vi "Untitled 1.vi"() -> ()   [LabVIEW 2018]
panel:
  in  "XYZAER":T1(array[cluster]) {"r" format="%1_6f"; "e" format="%1_6f"; "a" format="%1_6f"; "z" format="%1_6f"; "y" format="%1_6f"; "x" format="%1_6f"}
  out "Position Sensor Data":cluster{dbl, "x":sgl}[](graph)
  out "Tracker 1 - X,Y,Z":cluster{"x":sgl, "y":sgl, "z":sgl}(graph)
  out "Tracker 2 - X,Y,Z":cluster{"x":sgl, "y":sgl, "z":sgl}(graph)
  out "Tracker 3 - X,Y,Z":cluster{"x":sgl, "y":sgl, "z":sgl}(graph)
  out "Tracker 4 - X,Y,Z":cluster{"x":sgl, "y":sgl, "z":sgl}(graph)
  out "Connected":bool
  out "Start Time Text":string
  out "Stop Time Text":string
  out "Elapsed Time Text":string
  out "HostFrameCount":u32
  out "Running":bool
  out "Loop Iter":i32
  out "PnoData":bool
  in  "stop":bool
  out "error out":errorcluster {"code" format="%.0x"}
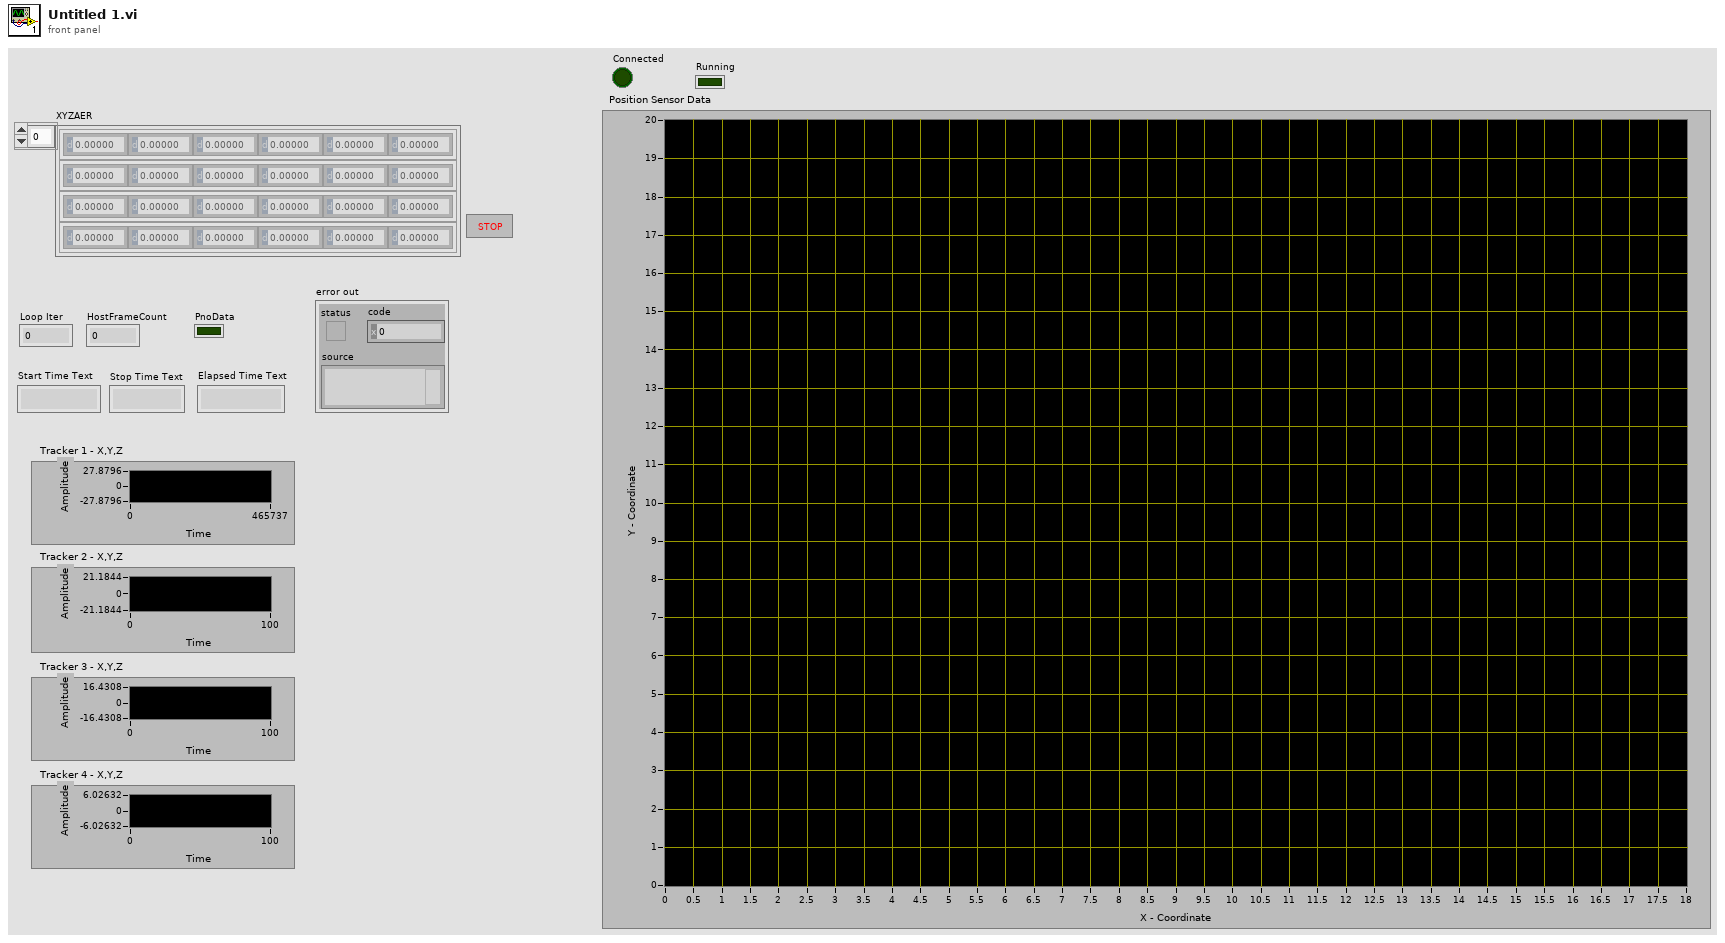
[diagram p1: front panel]
types:
  T1 = cluster{"x":sgl, "y":sgl, "z":sgl, "a":sgl, "e":sgl, "r":sgl}[]
  T2 = cluster{"x":sgl, "y":sgl, "z":sgl, "a":sgl, "e":sgl, "r":sgl}
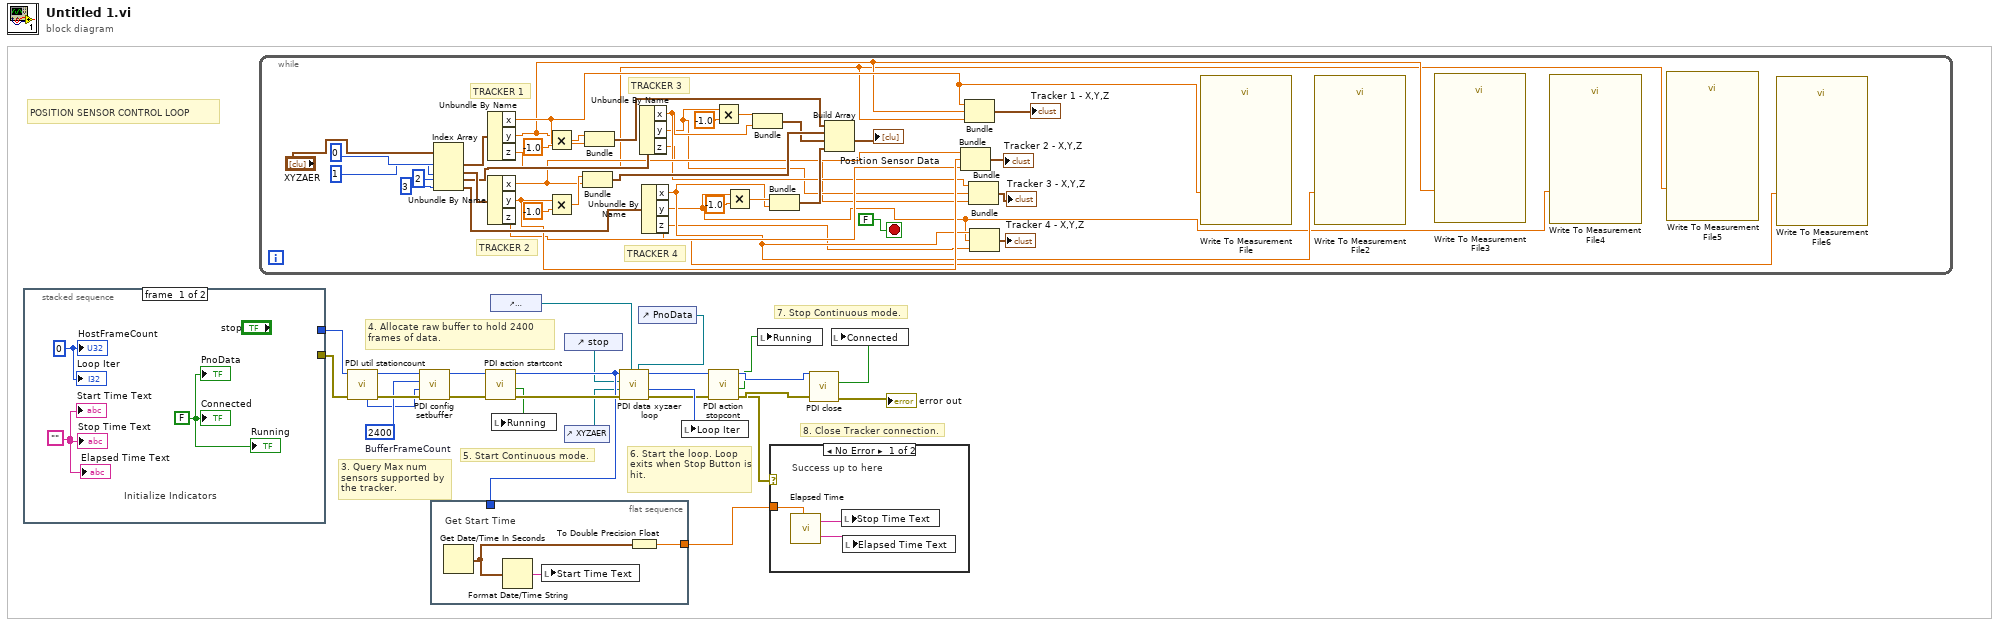
[diagram p0: block diagram]
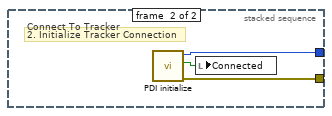
[diagram p3: hidden frame]
diagram:
  w3 = 2400  # BufferFrameCount
  # "POSITION SENSOR CONTROL LOOP"
  # "8. Close Tracker connection."
  # "3. Query Max num sensors supported by the tracker."
  # "4. Allocate raw buffer to hold 2400 frames of data."
  # "5. Start Continuous mode."
  # "7. Stop Continuous mode."
  # "6. Start the loop. Loop exits when Stop Button is hit."
  n1 = stacked-sequence {
    tunnel: [_ w30] -> w7
    tunnel: [_ w29] -> w6
    frame #0 {
      w25 = 0
      w26 = FALSE
      w27 = ""
      # "Initialize Indicators"
      "Connected" <- w26
      "Start Time Text" <- w27
      "Stop Time Text" <- w27
      "Elapsed Time Text" <- w27
      "HostFrameCount" <- w25
      "Running" <- w26
      "Loop Iter" <- w25
      "PnoData" <- w26
    }
    frame #1 {
      # "Connect To Tracker"
      # "2. Initialize Tracker Connection"
      n2 = call <instrlib>:"PDI initialize.vi"() -> ("error out"=w29:errorcluster, "Connected"=w28:bool, "pDev"=w30:u32)  [unwired: 1 in, 4 out]
      n3 = local write "Connected"(w28) -> ()
    }
  }
  n4 = while {
    stop <- FALSE stop-if-true
    # "TRACKER 4"
    # "TRACKER 3"
    # "TRACKER 2"
    # "TRACKER 1"
    n5 = Index Array(array="XYZAER", index #1=0 ("index"), index #2=1 ("index"), index #3=2 ("index"), index #4=3 ("index")) -> (element #1=w38:T2, element #2=w64:T2, element #3=w63:T2, element #4=w62:T2)
    n6 = Unbundle By Name(w38) -> ("x"=w36:sgl, "y"=w34:sgl, "z"=w32:sgl)
    n7 = Unbundle By Name(w64) -> ("x"=w48:sgl, "y"=w47:sgl, "z"=w46:sgl)
    n8 = Multiply(x=w34, y=sgl -1.0) -> (x*y=w56:sgl)
    n9 = Multiply(x=w47, y=-1.0) -> (x*y=w55:dbl)
    n10 = Bundle(w55, "x"=w48) -> (w51:cluster{dbl, "x":sgl})  [unwired: 1 in]
    n11 = Bundle(w56, "x"=w36) -> (w52:cluster{sgl, "x":sgl})  [unwired: 1 in]
    n12 = Unbundle By Name(w63) -> ("x"=w45:sgl, "y"=w44:sgl, "z"=w43:sgl)
    n13 = Unbundle By Name(w62) -> ("x"=w35:sgl, "y"=w33:sgl, "z"=w31:sgl)
    n14 = Multiply(x=w44, y=-1.0) -> (x*y=w54:dbl)
    n15 = Multiply(x=w33, y=-1.0) -> (x*y=w53:dbl)
    n16 = Bundle(w54, "x"=w45) -> (w50:cluster{dbl, "x":sgl})  [unwired: 1 in]
    n17 = Bundle(w53, "x"=w35) -> (w49:cluster{dbl, "x":sgl})  [unwired: 1 in]
    n18 = Build Array(w52, w51, w50, w49) -> (→"Position Sensor Data":cluster{dbl, "x":sgl}[])
    n19 = Bundle("x"=w48, "y"=w47, "z"=w46) -> (→"Tracker 2 - X,Y,Z":cluster{"x":sgl, "y":sgl, "z":sgl})  [unwired: 1 in]
    n20 = Bundle("x"=w36, "y"=w34, "z"=w32) -> (→"Tracker 1 - X,Y,Z":cluster{"x":sgl, "y":sgl, "z":sgl})  [unwired: 1 in]
    n21 = Bundle("x"=w45, "y"=w44, "z"=w43) -> (→"Tracker 3 - X,Y,Z":cluster{"x":sgl, "y":sgl, "z":sgl})  [unwired: 1 in]
    n22 = Bundle("x"=w35, "y"=w33, "z"=w31) -> (→"Tracker 4 - X,Y,Z":cluster{"x":sgl, "y":sgl, "z":sgl})  [unwired: 1 in]
    n23 = call "Write To Measurement File"("Signals"=w36) -> ()  [unwired: 16 in, 3 out]
    n24 = call "Write To Measurement File2"("Signals"=w35) -> ()  [unwired: 16 in, 3 out]
    n25 = call "Write To Measurement File3"("Signals"=w34) -> ()  [unwired: 16 in, 3 out]
    n26 = call "Write To Measurement File4"("Signals"=w33) -> ()  [unwired: 16 in, 3 out]
    n27 = call "Write To Measurement File5"("Signals"=w32) -> ()  [unwired: 16 in, 3 out]
    n28 = call "Write To Measurement File6"("Signals"=w31) -> ()  [unwired: 16 in, 3 out]
  }
  n29 = call <instrlib>:"PDI util stationcount.vi"("error in (no error)"=w6, "pDev"=w7) -> ("error out"=w5:errorcluster, "dup pDev"=w4:u32, "MaxCount"=w2:i32)  [unwired: 7 out]
  n30 = call <instrlib>:"PDI config setbuffer.vi"("error in (no error)"=w5, "Max sensors"=w2, "FrameCount"=w3, "pDev"=w4) -> ("error out"=w14:errorcluster, "dup pDev"=w15:u32)  [unwired: 6 out]
  n31 = flat-sequence {
    tunnel: w20 -> [_]
    tunnel: [w70] -> w16
    frame #0 {
      # "Get Start Time"
      n32 = Get Date/Time In Seconds() -> (seconds since 1Jan1904=w71:timestamp)
      n33 = Format Date/Time String(seconds (now)=w71) -> (date/time string=w72:string)  [unwired: 2 out]
      n34 = local write "Start Time Text"(w72) -> ()
      n35 = To Double Precision Float(number=w71) -> (double precision float=w70:dbl)
    }
  }
  n36 = call <instrlib>:"PDI action startcont.vi"("error in (no error)"=w14, "pDev"=w15) -> ("error out"=w21:errorcluster, "Running"=w13:bool, "dup pDev"=w20:u32)  [unwired: 7 out]
  n37 = control-ref of="HostFrameCount"() -> (w11:refnum<vi>)
  n38 = local write "Running"(w13) -> ()
  n39 = control-ref of="stop"() -> (w19:refnum<vi>)
  n40 = control-ref of="XYZAER"() -> (w10:refnum<vi>)
  n41 = control-ref of="PnoData"() -> (w1:refnum<vi>)
  n42 = call <instrlib>:"PDI data xyzaer loop.vi"("Data Ready Refnum"=w1, "FrameCount Ctl Ref"=w11, "error in (no error)"=w21, "xyzaer array\nRefnum"=w10, "Stop Ctl Ref"=w19, "pDev"=w20) -> ("error out"=w8:errorcluster, "Loop Iter"=w12:i32, "dup pDev"=w9:u32)  [unwired: 3 out]
  n43 = local write "Loop Iter"(w12) -> ()
  n44 = call <instrlib>:"PDI action stopcont.vi"("error in (no error)"=w8, "pDev"=w9) -> ("error out"=w17:errorcluster, "Running"=w22:bool, "dup pDev"=w23:u32)  [unwired: 7 out]
  n45 = local write "Running"(w22) -> ()
  n46 = case shown="No Error" w8 {
    tunnel: w16 -> [w73 _]
    frame No Error {
      # "Success up to here"
      n47 = call "Elapsed Time"("Set Start Time (s)"=w73) -> ("Present Text"=w75:string, "Elapsed Time Text"=w74:string)  [unwired: 4 in, 13 out]
      n48 = local write "Stop Time Text"(w75) -> ()
      n49 = local write "Elapsed Time Text"(w74) -> ()
    }
    frame Error {
      # "Error somewhere;\nStop Time is irrelevant"
    }
  }
  n50 = call <instrlib>:"PDI close.vi"("error in (no error)"=w17, "pDev"=w23) -> ("error out"=→"error out":errorcluster, "connected"=w18:bool)  [unwired: 8 out]
  n51 = local write "Connected"(w18) -> ()
